vi "Base Init.vi"(10 "Is Sync":bool) -> (2 "Sender":refnum<class "Sender.lvclass">)   [LabVIEW 2020, in "jettl.lvlib" / "Sender.lvlib"]
uses:
  Sender.lvlib
  Base Sender/Base Sender.lvclass
  Sender/Sender.lvclass
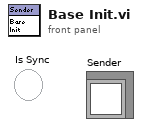
[diagram p1: front panel]
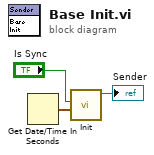
[diagram p0: block diagram]
diagram:
  n1 = Get Date/Time In Seconds() -> (seconds since 1Jan1904=w2:timestamp)
  n2 = call "Init.vi"("Time"=w2, "Is Sync"="Is Sync") -> ("Base Sender out"=→"Sender":refnum<class "Base Sender.lvclass">)  [unwired: 9 in]
